vi "W2E1.vi"() -> ()   [LabVIEW 2023]
panel:
  in  "Numeric":dbl
  out "Numeric 3":i32
  out "Numeric 2":dbl
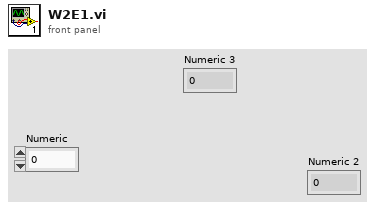
[diagram p1: front panel]
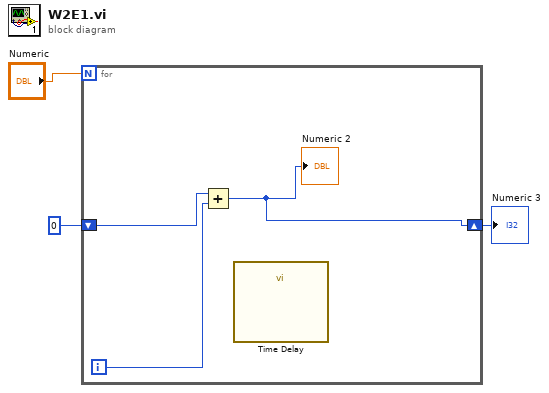
[diagram p0: block diagram]
diagram:
  n1 = for {
    N: "Numeric" -> [_]
    shift-right: [w4] -> w2
    shift-left: 0 -> [w6]
    i -> [w5]
    n2 = Add(x=w6, y=w5) -> (x+y=w4:i32)
    "Numeric 2" <- w4
    n3 = call "Time Delay"() -> ()  [unwired: 11 in, 1 out]
  }
  "Numeric 3" <- w2
